vi "Moneda 2.vi"(8 "error in (no error)":errorcluster, 11 "Monedas in":refnum<class "Monedas.lvclass">) -> (0 "error out":errorcluster, 3 "Monedas out":refnum<class "Monedas.lvclass">)   [LabVIEW 2020, in "Monedas.lvlib" / "Monedas.lvclass"]
uses:
  Monedas.lvclass
  Monedas.lvclass/Monedas.ctl
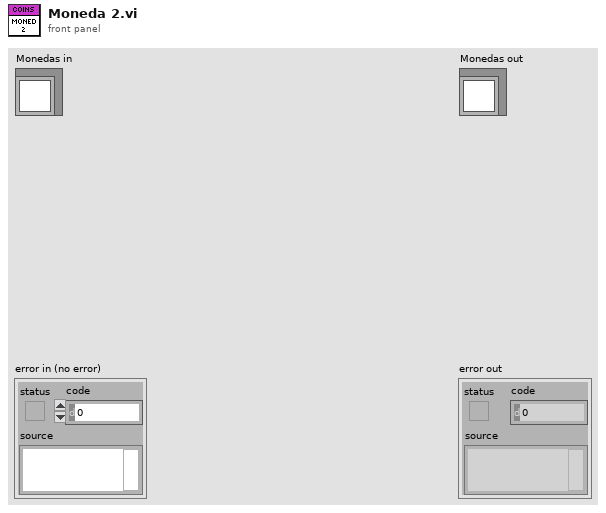
[diagram p1: front panel]
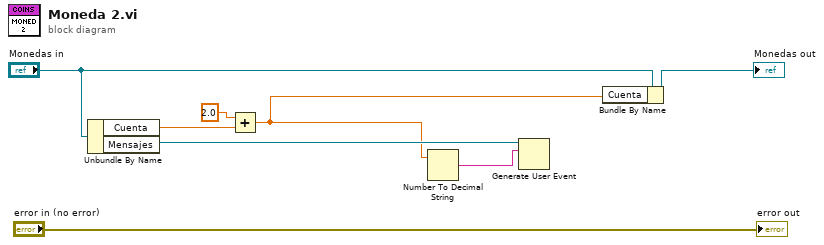
[diagram p0: block diagram]
diagram:
  n1 = Unbundle By Name("Monedas in") -> ("Cuenta"=w4:dbl, "Mensajes"=w3:refnum<user-event>)
  n2 = Add(x=2.0, y=w4) -> (x+y=w2:dbl)
  n3 = Number To Decimal String(number=w2) -> (decimal integer string=w1:string)  [unwired: 1 in]
  n4 = Generate User Event(user event=w3, event data cluster=w1) -> ()  [unwired: 2 in, 2 out]
  n5 = Bundle By Name(cluster="Monedas in", "Cuenta"=w2) -> (→"Monedas out":refnum<class "Monedas.lvclass">)
  "error out" <- "error in (no error)"
